vi "armCalculator.vi"(3 "AIDeviceRef":T1={"DevStatus"={"status"=FALSE, "code"=0, "source"=""}, "Controller"=enum."Controller 1", "Analog Channel"=enum."AI 1"}) -> (0 "Scaled Pot Val":dbl)   [LabVIEW 2014]
uses:
  <vilib>/Rock Robotics/WPI/AnalogChannel/WPI_AnalogChannelDevRef.ctl
  <vilib>/Rock Robotics/SystemInterfaces/Typedef/FPGA_TypedefAnalogModule.ctl
  <vilib>/Rock Robotics/SystemInterfaces/AI/FPGA_AIChannel.ctl
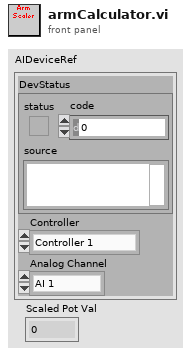
[diagram p1: front panel]
types:
  T1 = typedef "WPI_AnalogChannelDevRef.ctl" = cluster{"DevStatus":errorcluster, "Controller":T2, "Analog Channel":T3}
  T2 = typedef "FPGA_TypedefAnalogModule.ctl" = enum16{"Controller 1"}
  T3 = typedef "FPGA_AIChannel.ctl" = enum8{"AI 0", "AI 1", "AI 2", "AI 3", "AI MXP 0", "AI MXP 1", "AI MXP 2", "AI MXP 3", "Invalid"}
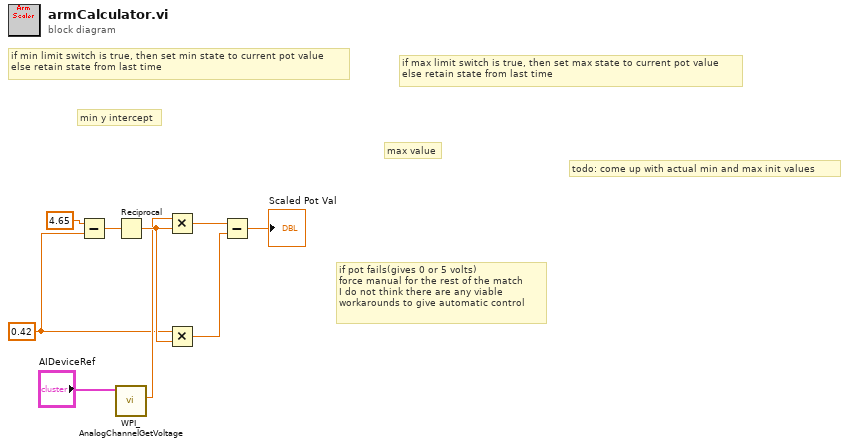
[diagram p0: block diagram]
diagram:
  w2 = 0.42
  # "if pot fails(gives 0 or 5 volts)\nforce manual for the rest of the match\nI do not think there are any viable\nworkarounds to give automatic control"
  # "todo: come up with actual min and max init values"
  # "if max limit switch is true, then set max state to current pot value\nelse retain state from last time"
  # "if min limit switch is true, then set min state to current pot value\nelse retain state from last time"
  # "max value"
  # "min y intercept"
  n1 = Subtract(x=4.65 ("Voltage"), y=w2) -> (x-y=w8:dbl)
  n2 = Reciprocal(x=w8) -> (1/x=w5:dbl)
  n3 = call <vilib>:"WPI_AnalogChannelGetVoltage.vi"("AIDeviceRef"="AIDeviceRef") -> ("Voltage"=w3:dbl)  [unwired: 8 in, 2 out]
  n4 = Multiply(x=w3, y=w5) -> (x*y=w7:dbl)
  n5 = Multiply(x=w2, y=w5) -> (x*y=w4:dbl)
  n6 = Subtract(x=w7, y=w4) -> (x-y=→"Scaled Pot Val":dbl)
